vi "SaveFile.vi"(8 "error in (no error)":errorcluster, 11 "aparCfg in":refnum<class "aparCfg.lvclass">) -> (0 "error out":errorcluster, 3 "aparCfg out":refnum<class "aparCfg.lvclass">)   [LabVIEW 2019, in "aparCfg.lvclass"]
uses:
  aparCfg.lvclass
  aparConfig.ctl
  N5222A PNA/N5222AConfig.ctl
  ArrayController/ACConfig.ctl
  Datalog/DataLogConfig.ctl
  aparCfg.lvclass/aparCfg.ctl
panel:
  out "apar properties":T1={"N5222AConfig"={"ResourceName"="", "Enable"=FALSE, "Channel"=1, "CalFileName"="", "MeasName"="", "TempDatFile"="", "Power, dBm"=-30.0, "NumPoints"=201, "Start Freq, Hz"=5000000000.0, "Stop Freq, Hz"=6000000000.0, "NumAverages"=20, "Sweep Type"=0, "IF Bandwidth"=0.0}, "ACConfig"={"Board 1 alias"="192.168.1.110", "Board 1 Enable"=FALSE, "Board 2 alias"="192.168.1.110", "Board 2 Enable"=FALSE}, "DataLogConfig"={"FilePath"=path ""}} {"N5222AConfig"."Sweep Type" items=["Linear Frequency", "Log Frequency", "Power Sweep", "CW Time"]; "N5222AConfig"."Stop Freq, Hz" format="%_3p"; "N5222AConfig"."Start Freq, Hz" format="%_3p"}
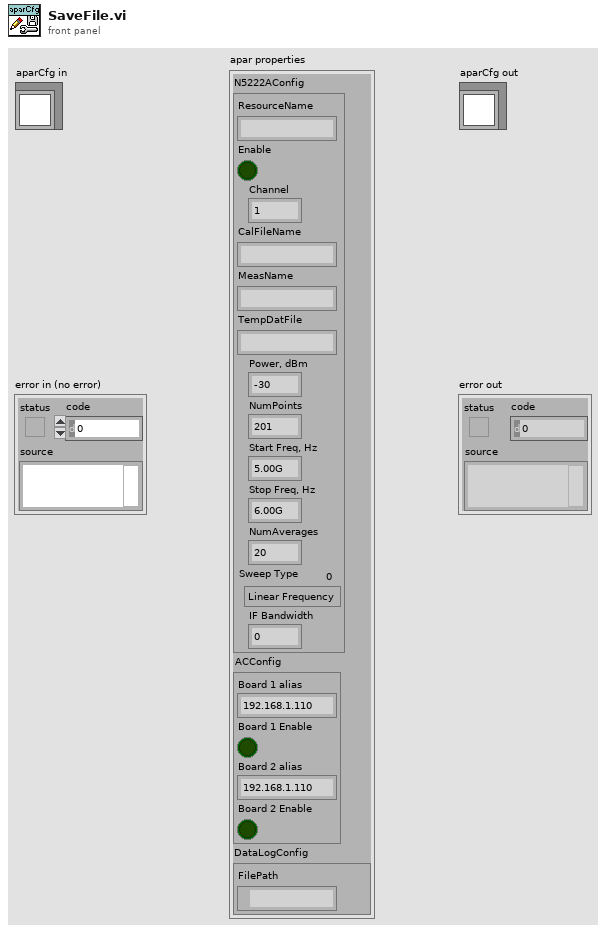
[diagram p1: front panel]
types:
  T1 = typedef "aparCfg.lvclass/aparConfig.ctl" = cluster{"N5222AConfig":T2, "ACConfig":T3, "DataLogConfig":T4}
  T2 = typedef "N5222AConfig.ctl" = cluster{"ResourceName":string, "Enable":bool, "Channel":i32, "CalFileName":string, "MeasName":string, "TempDatFile":string, "Power, dBm":dbl, "NumPoints":i32, "Start Freq, Hz":dbl, "Stop Freq, Hz":dbl, "NumAverages":i32, "Sweep Type":i32, "IF Bandwidth":dbl}
  T3 = typedef "ACConfig.ctl" = cluster{"Board 1 alias":string, "Board 1 Enable":bool, "Board 2 alias":string, "Board 2 Enable":bool}
  T4 = typedef "DataLogConfig.ctl" = cluster{"FilePath":path}
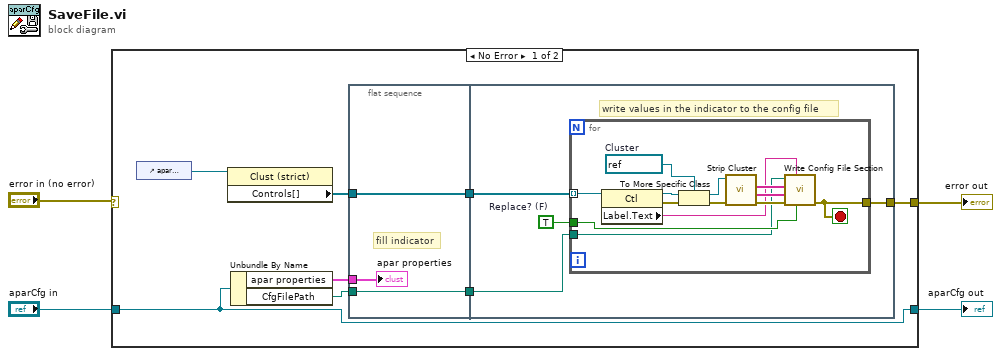
[diagram p0: block diagram]
diagram:
  n1 = case shown="No Error" "error in (no error)" {
    selector: "error in (no error)" -> [_ w34]
    tunnel: [w6 w34] -> w1
    tunnel: [w7 w33] -> w2
    tunnel: "aparCfg in" -> [w7 w33]
    frame No Error {
      n2 = control-ref of="apar properties"() -> (w5:refnum<vi>)
      n3 = property class="Clust (strict)"(reference=w5) -> ("Controls[]"=w10:refnum<vi>[])  [unwired: 1 in, 2 out]
      n4 = Unbundle By Name(w7) -> ("apar properties"=w8:T1, "CfgFilePath"=w9:path)
      n5 = flat-sequence {
        tunnel: w8 -> [w13]
        tunnel: w9 -> [w15]
        tunnel: [w15] -> w12
        tunnel: [w14] -> w11
        tunnel: w10 -> [w14]
        tunnel: w12 -> [w16]
        tunnel: w11 -> [w18]
        tunnel: [w17] -> w6
        frame #0 {
          # "fill indicator"
          "apar properties" <- w13
        }
        frame #1 {
          w19 = TRUE  # Replace? (F)
          # "write values in the indicator to the config file"
          n6 = for {
            tunnel: [w26] -> w17
            tunnel: w19 -> [w23]
            tunnel: w16 -> [w22]
            tunnel: w18 -> [w21] mode=indexing
            stop <- w26 stop-if-true
            w32 = refnum<vi> refnum  # Cluster
            n7 = property class="Ctl"(reference=w21) -> (reference out=w25:refnum<vi>, error out=w20:errorcluster, "Label.Text"=w24:string)  [unwired: 1 in]
            n8 = To More Specific Class(target class=w32, reference=w25, error in=w20) -> (specific class reference=w31:refnum<vi>, error out=w28:errorcluster)
            n9 = call "Strip Cluster.vi"("error in (no error)"=w28, "Cluster Refnum"=w31) -> ("error out"=w27:errorcluster, "Values"=w29:string[], "Keys"=w30:string[])  [unwired: 6 in, 1 out]
            n10 = call "Write Config File Section.vi"("Replace? (F)"=w23, "Section"=w24, "error in"=w27, "Values"=w29, "Keys"=w30, "INI path"=w22) -> ("error out"=w26:errorcluster)  [unwired: 5 in]
          }
        }
      }
    }
    frame Error {
    }
  }
  "error out" <- w1
  "aparCfg out" <- w2
